vi "set_config_cluster.vi"(8 "error in (no error)":errorcluster, 10 "config cluster variant":variant, 11 "TrajectoryDL090201FrameScan in":refnum<class "TrajectoryDL090201FrameScan.lvclass">) -> (0 "error out":errorcluster, 3 "TrajectoryDL090201FrameScan out":refnum<class "TrajectoryDL090201FrameScan.lvclass">)   [LabVIEW 2010, in "TrajectoryDL090201FrameScan.lvclass"]
uses:
  TrajectoryDL090201FrameScan.lvclass
  TrajectoryDL090201FrameScan.lvclass/TrajectoryDL090201FrameScan.ctl
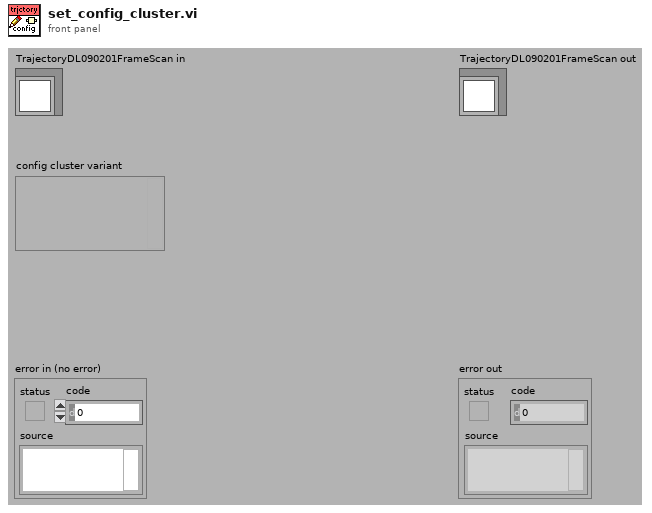
[diagram p1: front panel]
types:
  T1 = typedef "TrajectoryDL090201FrameScan.lvclass/config_cluster.ctl" = cluster{"x scan cut-off fraction":dbl, "x retrace fraction":dbl, "y retrace fraction":dbl}
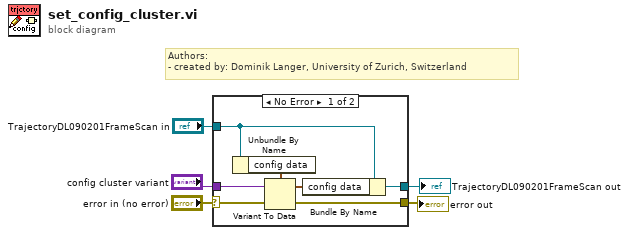
[diagram p0: block diagram]
diagram:
  # "Authors: \n- created by: Dominik Langer, University of Zurich, Switzerland"
  n1 = case shown="No Error" "error in (no error)" {
    selector: "error in (no error)" -> [w10 w13]
    tunnel: "TrajectoryDL090201FrameScan in" -> [w8 w14]
    tunnel: [w7 w13] -> w4
    tunnel: [w6 w14] -> w1
    tunnel: "config cluster variant" -> [w9 _]
    frame No Error {
      n2 = Unbundle By Name(w8) -> ("config data"=w12:T1)
      n3 = Variant To Data(error in=w10, Variant=w9, type=w12) -> (error out=w7:errorcluster, data=w11:T1)
      n4 = Bundle By Name(cluster=w8, "config data"=w11) -> (w6:refnum<class "TrajectoryDL090201FrameScan.lvclass">)
    }
    frame Error {
    }
  }
  "error out" <- w4
  "TrajectoryDL090201FrameScan out" <- w1
